vi "VI Server_TREE_Items_SET.vi"(6 "Column Header Strings[]":T1[](array[typedef]), 7 "Label":string, 8 "error in":errorcluster, 9 "Tree.Ref":refnum<vi>, 10 "SingleInstance":bool=TRUE, 11 "VI Server.RefsCluster":T2) -> (0 "error out":errorcluster, 1 "Tree.Ref":refnum<vi>, 3 "VI Server.RefsCluster.DUP":T2)   [LabVIEW 2020]
uses:
  VI Server_TypeDefs/VI Server_RefsCluster.ctl
  VI Server_TypeDefs/VI Server_Tree_Items.ctl
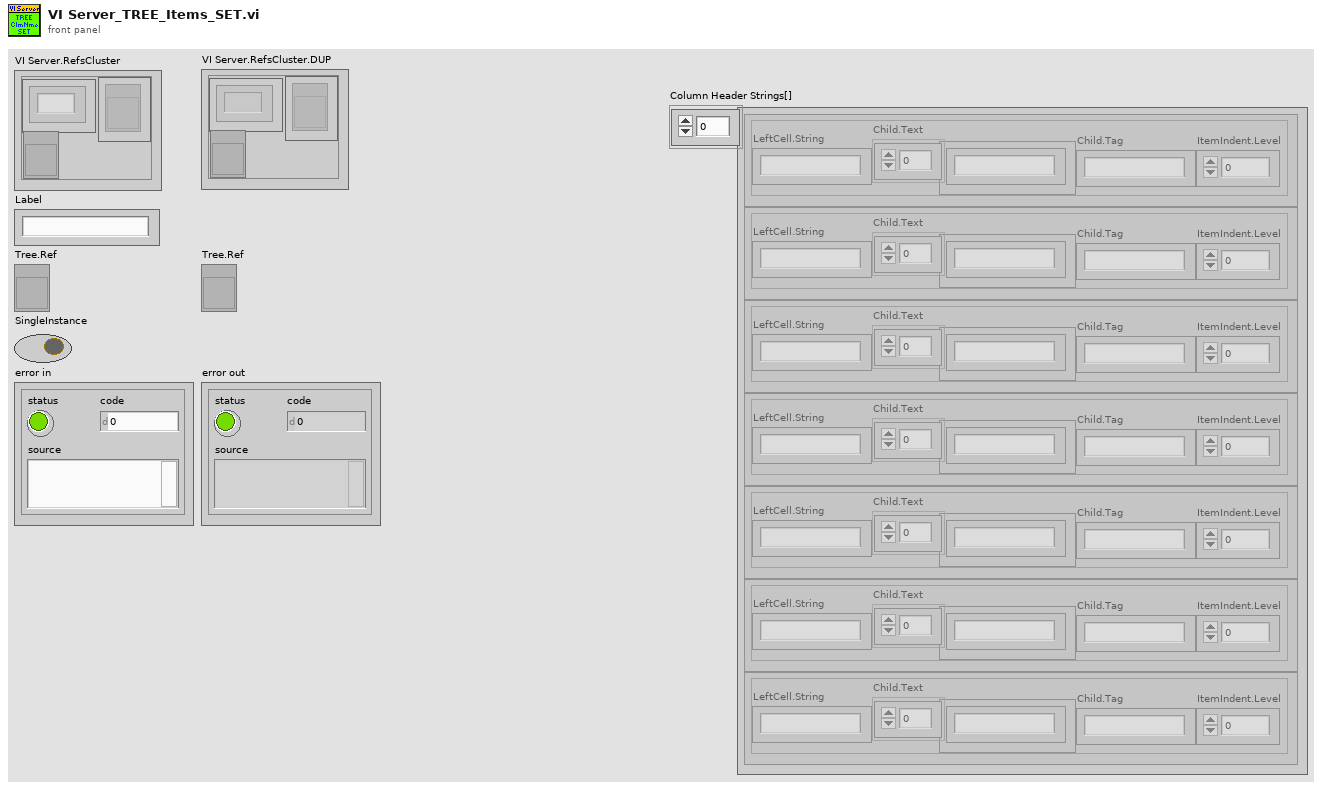
[diagram p1: front panel]
types:
  T1 = typedef "VI Server_Tree_Items.ctl" = cluster{"LeftCell.String":string, "Child.Text":string[], "Child.Tag":string, "ItemIndent.Level":i32}
  T2 = typedef "VI Server_RefsCluster.ctl" = cluster{"Labels":string[], "Refs":refnum<vi>[], "VI Ref":refnum<vi>}
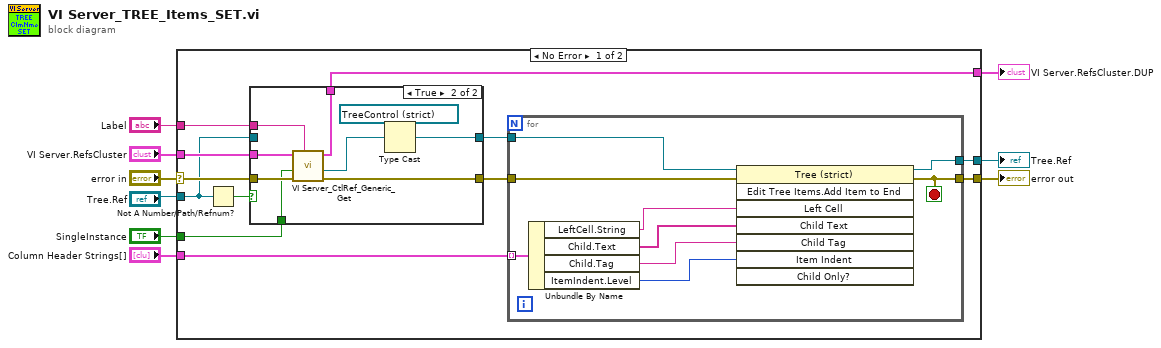
[diagram p0: block diagram]
diagram:
  n1 = case shown="No Error" "error in" {
    selector: "error in" -> [w21 w44]
    tunnel: [w14 w44] -> w8
    tunnel: "VI Server.RefsCluster" -> [w20 w43]
    tunnel: [w19 w43] -> w6
    tunnel: "Label" -> [w18 _]
    tunnel: "SingleInstance" -> [w17 _]
    tunnel: [w13 _] -> w2
    tunnel: "Column Header Strings[]" -> [w12 _]
    tunnel: "Tree.Ref" -> [w10 _]
    frame No Error {
      n2 = Not A Number/Path/Refnum?(number/path/refnum=w10) -> (NaN/Path/Refnum?=w11:bool)
      n3 = case shown="True" w11 {
        tunnel: w21 -> [w22 w33]
        tunnel: w20 -> [w24 w32]
        tunnel: [w24 w31] -> w19
        tunnel: w18 -> [_ w30]
        tunnel: w17 -> [_ w28]
        tunnel: [w23 w26] -> w16
        tunnel: [w22 w25] -> w15
        tunnel: w10 -> [w23 _]
        frame False {
        }
        frame True {
          n4 = call "VI Server_CtlRef_Generic_Get.vi"("Control.Label"=w30, "error in"=w33, "SingleInstance"=w28, "VI Server.RefsCluster"=w32) -> ("error out"=w25:errorcluster, "Control.Ref.Generic"=w29:refnum<vi>, "VI Server.RefsCluster.DUP"=w31:T2)  [unwired: 5 in]
          n5 = Type Cast(type=refnum<vi> refnum ("Tree"), x=w29) -> (*(type *) &x=w26:refnum<vi>)
        }
      }
      n6 = for {
        tunnel: w15 -> [w41]
        tunnel: [w39] -> w14
        tunnel: w16 -> [w42]
        tunnel: [w40] -> w13
        tunnel: w12 -> [w38] mode=indexing
        stop <- w39 stop-if-true
        n7 = Unbundle By Name(w38) -> ("LeftCell.String"=w37:string, "Child.Text"=w36:string[], "Child.Tag"=w35:string, "ItemIndent.Level"=w34:i32)
        n8 = invoke on="Invoke Node" class="Tree (strict)" method="Edit Tree Items.Add Item to End"(reference=w42, error in=w41, "Left Cell"=w37, "Child Text"=w36, "Child Tag"=w35, "Item Indent"=w34) -> (reference out=w40:refnum<vi>, error out=w39:errorcluster)  [unwired: 2 in, 6 out]
      }
    }
    frame Error {
    }
  }
  "VI Server.RefsCluster.DUP" <- w6
  "error out" <- w8
  "Tree.Ref" <- w2
